vi "displayData.vi"() -> ()   [LabVIEW 2017]
panel:
  in  "dataToRead":u32
  out "size(s) 2":i32
  out "size(s)":i32[](array[numeric])
  out "Waveform Graph":i16[](graph)
  in  "ArrayOut":i16[][](array[numeric])
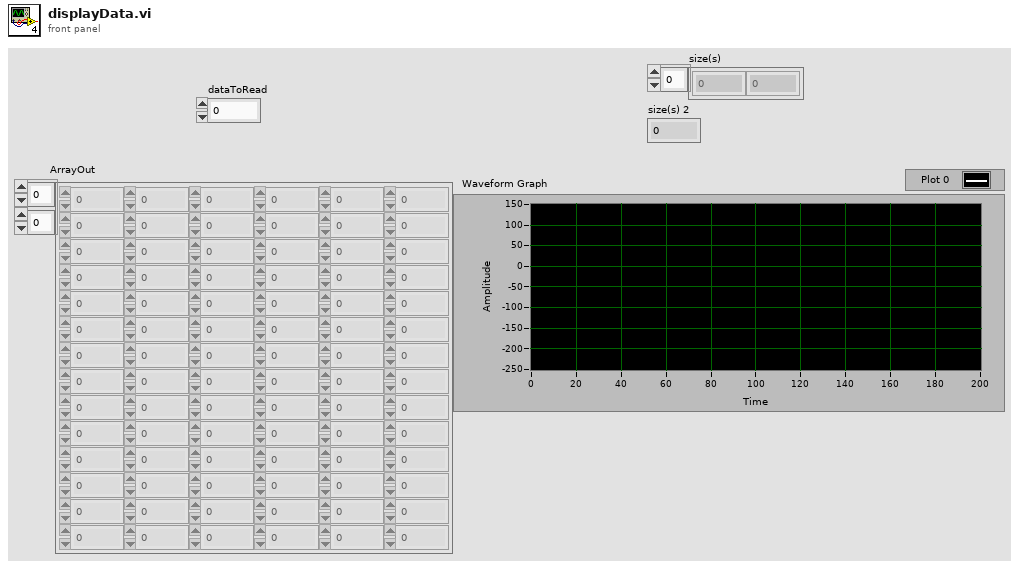
[diagram p1: front panel]
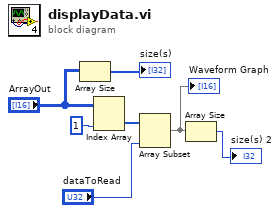
[diagram p0: block diagram]
diagram:
  n1 = Array Size(array="ArrayOut") -> (size(s)=→"size(s)":i32[])
  n2 = Index Array(array="ArrayOut", index (col)=1 ("disabled index (col)")) -> (element=w3:i16[])  [unwired: 1 in]
  n3 = Array Subset(array=w3, length="dataToRead") -> (w1:i16[])  [unwired: 1 in]
  "Waveform Graph" <- w1
  n4 = Array Size(array=w1) -> (size(s)=→"size(s) 2":i32)
